vi "Lockin.DAQ.TestLauncher.vi"() -> ()   [LabVIEW 2019, in "Lockin.DAQ.lvclass"]
uses:
  Lockin.DAQ.lvclass
  <vilib>/JKI/JKI SMO/SMO/SMO.lvclass
  <vilib>/JKI/JKI SMO/SMO/Typedefs/SMOState --Enum.ctl
  Typedefs/Set State-enum.ctl
  Instrument.Lockin/Instrument.Lockin.lvclass
  C:/Program Files (x86)/National Instruments/LabVIEW 2016/vi.lib/JKI/JKI SMO/SMO/SMO.lvclass
  Instrument.Lockin/Typedefs/Results Type--Enum.ctl
  Typedefs/Function-enum.ctl
  Typedefs/AO-cluster.ctl
  Typedefs/REF-cluster.ctl
  Typedefs/446xAO-enum.ctl
  Typedefs/AO.config(UI)-cluster.ctl
  Typedefs/AO.config(UI)-array.ctl
  Typedefs/AI.coupling-enum.ctl
  Typedefs/446xAI-enum.ctl
  Typedefs/AI.config(UI)-cluster.ctl
  Typedefs/AI.config(UI)-array.ctl
  Typedefs/Sampling.ctl
  Typedefs/Sample Mode--Ring.ctl
  Typedefs/State-enum.ctl
  Instrument.Lockinl.UI/Typedefs/REF Channel--Cluster.ctl
  Instrument.Lockinl.UI/Instrument.Lockin.UI.lvclass
  Instrument.Lockinl.UI/Typedefs/AO Channel--Cluster.ctl
panel:
  out "DAQ state":T1=enum."created"
  in  "Tab Control 2":T2(tab)=enum."AI"
  out "AO":waveform(dbl)[](graph)
  out "AI":waveform(dbl)[](graph)
  out "WFM 3":waveform(dbl)[](graph)
  out "REF":waveform(dbl)[](graph)
  out "Results":dbl[](graph)
  in  "Reset DAQ":bool
  in  "Stop DAQ":bool
  in  "Start DAQ":bool
  in  "Tab Control":enum32{"Output", "REF", "DAQ"}(tab)=enum."DAQ"
  in  "Channels: AO":T3 {"Phase" format="%.3g"; "Frequency" min=0.0001 max=10000.0 format="%.3g"; "Offset" format="%.3p"; "Amplitude" min=0.0 max=10.0 format="%.3p"}
  in  "Channels: Lockin":T6=[{"Enable?"=FALSE, "Channel"=13, "Frequency"=0.1, "Phase"=0.0, "TC"=1e-05, "Roll-Off"=1}] {"Roll-Off" min=1; "TC" min=0.0001 format="%#_3p"; "Phase" format="%.3g"; "Frequency" min=0.0001 max=10000.0 format="%.3g"}
  in  "Gain":dbl[](array[numeric])=[1.0, 1.0]
  in  "AO Configuration":T8=[{"AO.Range"=enum."±0.1", "AO.channels"="PXI1Slot2/ao0:1"}]
  in  "AI Configuration":T11=[{"AI.Coupling"=10050, "AI.channels"="PXI1Slot2/ai0:1", "AI.Range"=enum."±0.316"}] {"AI.Coupling" items=["AC"=10045, "DC"=10050, "GND"=10066]}
  in  "sampling":T15={"Fs"=204789.0, "#s"=15753}
  in  "sample mode":T16=10123 items=["Finite Samples"=10178, "Continuous Samples"=10123]
  out "SMO State":T17=enum."Stopped"
  out "error out":errorcluster
  in  "Stop":bool
  # "Basic SMO Test Launcher"
  # "For instructions on how to use the JKI State Machine Objects, examples and video tutorials, visit:\nhttp://jki.net/state-machine-objects/\n\nJKI State Machine Objects™\nhttp://jki.net/state-machine-objects/\nCopyright (C) 2005-2015, JKI <info@jki.net>\nALL RIGHTS RESERVED"
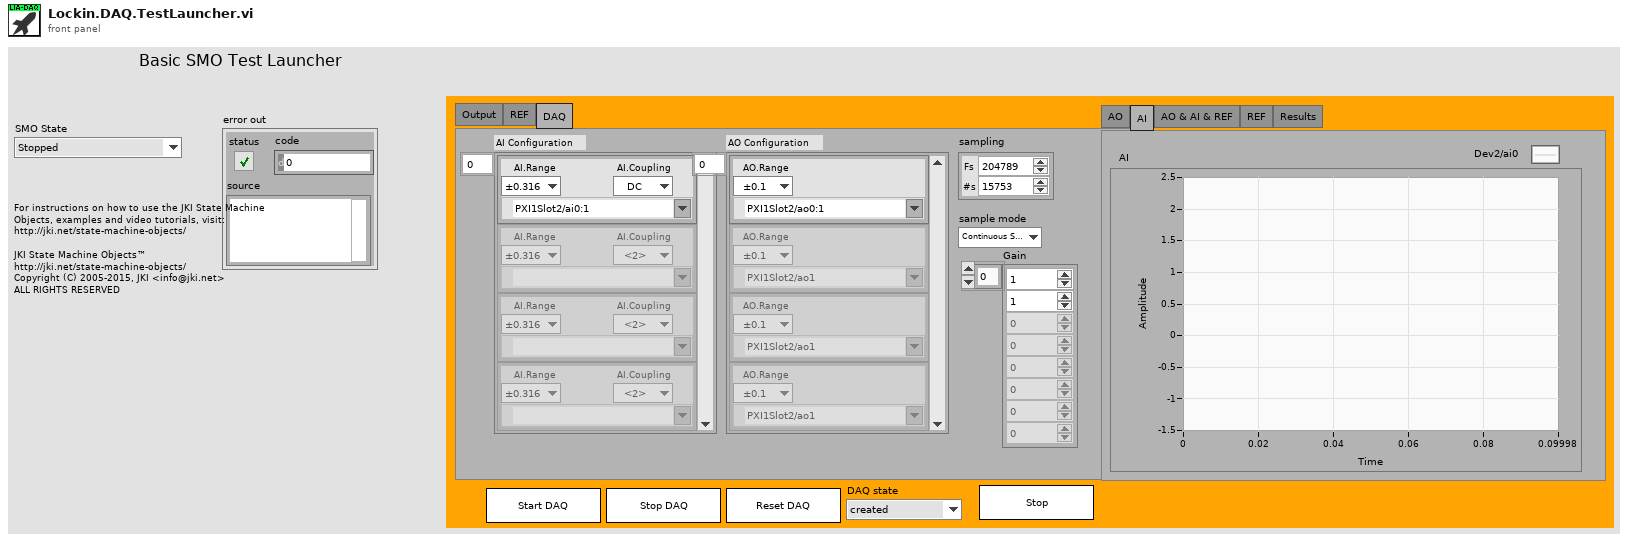
[diagram p1: front panel]
types:
  T1 = typedef "Lockin.DAQ.lvclass/State-enum.ctl" = enum16{"idle", "created", "started", "stopped", "sweeping"}
  T2 = enum32{"AO", "AI", "AO & AI & REF", "REF", "Results"}
  T3 = typedef "Lockin.DAQ.lvclass/AO-cluster.ctl" = T4[]
  T4 = typedef "Instrument.Lockin.UI.lvclass/AO Channel--Cluster.ctl" = cluster{"Enable?":bool, "Channel":i32, "Amplitude":dbl, "Offset":dbl, "Frequency":dbl, "Phase":dbl, "Function":T5, "Sweeping?":bool}
  T5 = typedef "Lockin.DAQ.lvclass/Function-enum.ctl" = enum16{"Sine", "Triangle", "Square"}
  T6 = typedef "Lockin.DAQ.lvclass/REF-cluster.ctl" = T7[]
  T7 = typedef "Instrument.Lockin.UI.lvclass/REF Channel--Cluster.ctl" = cluster{"Enable?":bool, "Channel":i32, "Frequency":dbl, "Phase":dbl, "TC":dbl, "Roll-Off":i32}
  T8 = typedef "Lockin.DAQ.lvclass/AO.config(UI)-array.ctl" = T9[]
  T9 = typedef "Lockin.DAQ.lvclass/AO.config(UI)-cluster.ctl" = cluster{"AO.Range":T10, "AO.channels":tag}
  T10 = typedef "Lockin.DAQ.lvclass/446xAO-enum.ctl" = enum16{"±0.1", "±1.0", "±10.0"}
  T11 = typedef "Lockin.DAQ.lvclass/AI.config(UI)-array.ctl" = T12[]
  T12 = typedef "Lockin.DAQ.lvclass/AI.config(UI)-cluster.ctl" = cluster{"AI.Coupling":T13, "AI.channels":tag, "AI.Range":T14}
  T13 = typedef "Lockin.DAQ.lvclass/AI.coupling-enum.ctl" = u16
  T14 = typedef "Lockin.DAQ.lvclass/446xAI-enum.ctl" = enum16{"±0.316", "±1.00", "±3.16", "±10.0", "±31.6", "±42.4"}
  T15 = typedef "Lockin.DAQ.lvclass/Sampling.ctl" = cluster{"Fs":dbl, "#s":i32}
  T16 = typedef "Lockin.DAQ.lvclass/Sample Mode--Ring.ctl" = i32
  T17 = typedef "SMO.lvclass/SMOState --Enum.ctl" = enum16{"unknown", "Created", "Started", "Stopped"}
  T18 = typedef "SMO.lvclass/Public Events.ctl" = cluster{"Error":refnum<user-event>, "State":refnum<user-event>, "Reserve State":refnum<user-event>}
  T19 = typedef "Lockin.DAQ.lvclass/PublicEvents--Cluster.ctl" = cluster{"getAO":refnum<user-event>, "getAI":refnum<user-event>, "getREF":refnum<user-event>, "getResults":refnum<user-event>, "getCalibration":refnum<user-event>, "getAOChannels":refnum<user-event>, "getREFChannels":refnum<user-event>, "getDAQState":refnum<user-event>, "getSweepResults":refnum<user-event>, "getSweepWaveforms":refnum<user-event>, "getDAQconfig":refnum<user-event>}
  T20 = cluster{"Event Registration Refnum":refnum<event-registration>}
  T21 = typedef "Lockin.DAQ.lvclass/Set State-enum.ctl" = enum16{"start", "stop", "reset", "start sweep", "stop sweep"}
  T22 = typedef "Instrument.Lockin.lvclass/Results Type--Enum.ctl" = enum16{"X", "Y", "R", "Theta", "Mean"}
  T23 = typedef "Lockin.DAQ.lvclass/AI.config-array.ctl" = T24[]
  T24 = typedef "Lockin.DAQ.lvclass/AI.config-cluster.ctl" = cluster{"AI.channels":tag, "AI.Coupling":T13, "AI.Range":T14, "input terminal configuration":i32, "DAQ Type":T25}
  T25 = typedef "Lockin.DAQ.lvclass/DAQType-enum.ctl" = enum16{"None", "USB 4431", "PXI 446x"}
  T26 = typedef "Lockin.DAQ.lvclass/AO.config-array.ctl" = T27[]
  T27 = typedef "Lockin.DAQ.lvclass/AO.config-cluster.ctl" = cluster{"AO.channels":tag, "AO.Range":T10, "output terminal configuration":i32, "DAQ Type":T25}
  T28 = typedef "Lockin.DAQ.lvclass/PublicEvents--Lockin.DAQ.getAO.ctl" = waveform(dbl)[]
  T29 = typedef "Lockin.DAQ.lvclass/PublicEvents--Lockin.DAQ.getAI.ctl" = waveform(dbl)[]
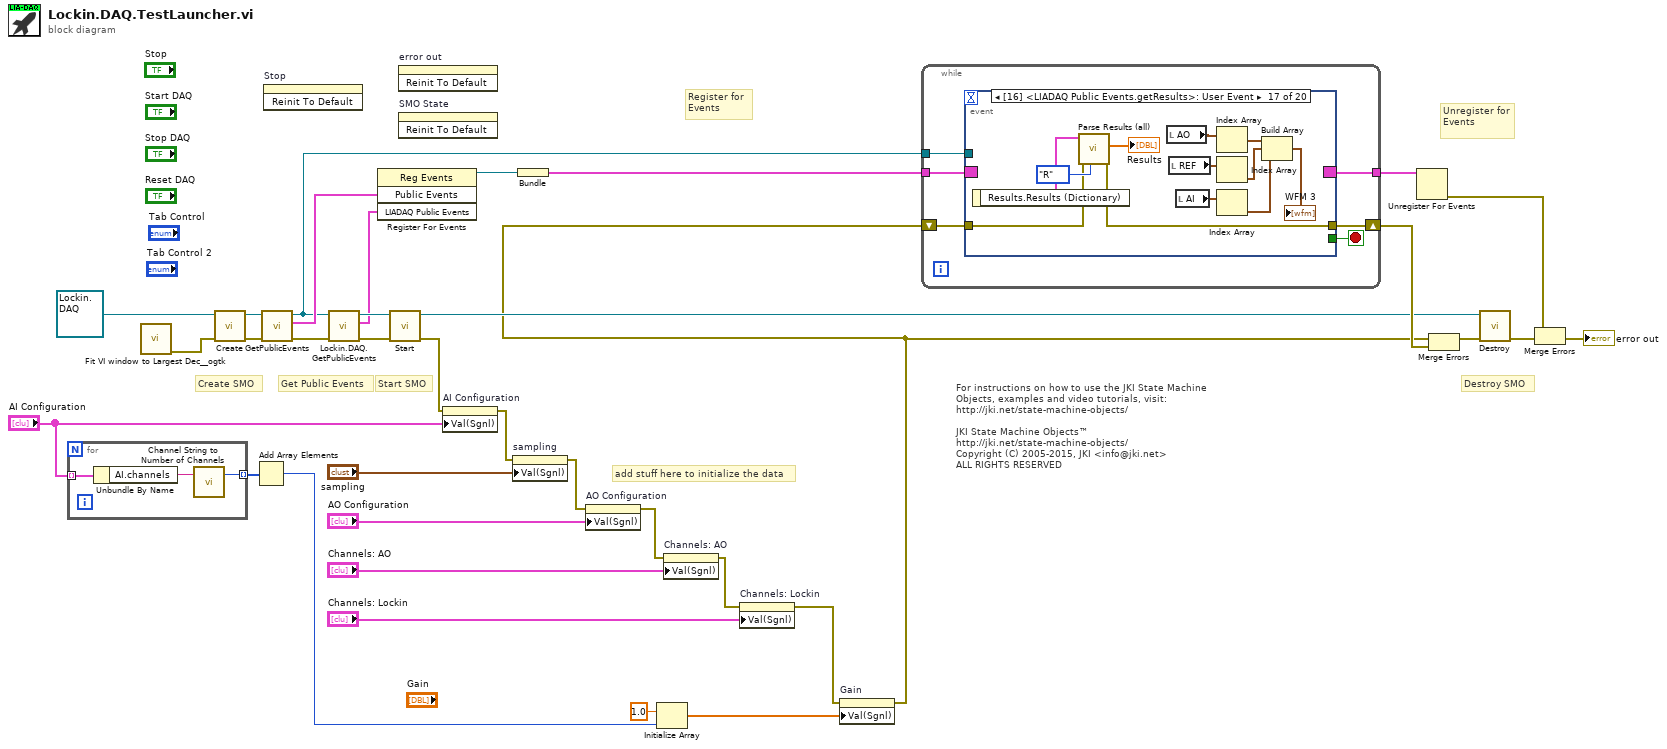
[diagram p0: block diagram]
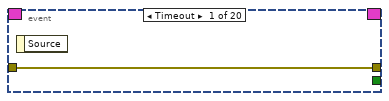
[diagram p2: hidden frame]
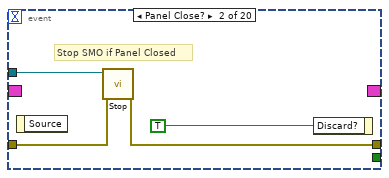
[diagram p3: hidden frame]
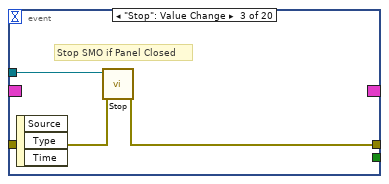
[diagram p4: hidden frame]
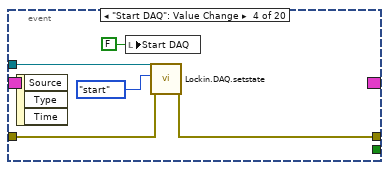
[diagram p5: hidden frame]
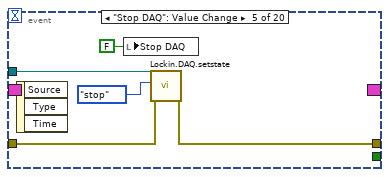
[diagram p6: hidden frame]
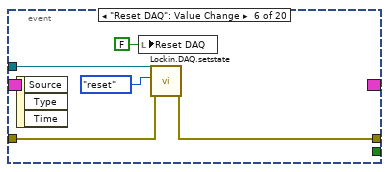
[diagram p7: hidden frame]
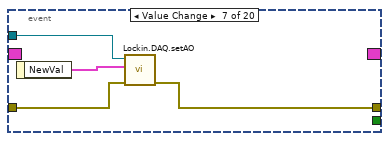
[diagram p8: hidden frame]
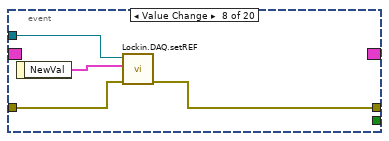
[diagram p9: hidden frame]
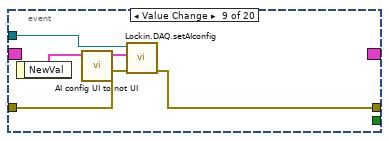
[diagram p10: hidden frame]
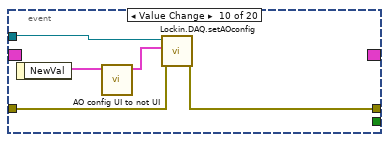
[diagram p11: hidden frame]
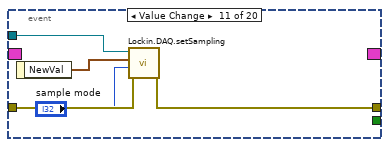
[diagram p12: hidden frame]
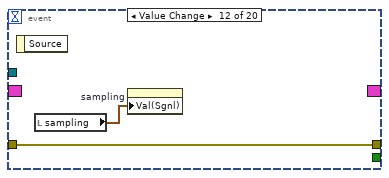
[diagram p13: hidden frame]
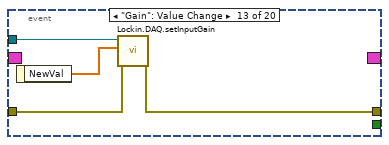
[diagram p14: hidden frame]
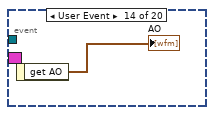
[diagram p15: hidden frame]
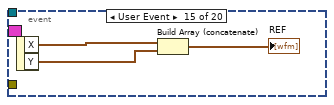
[diagram p16: hidden frame]
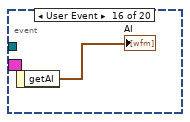
[diagram p17: hidden frame]
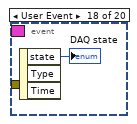
[diagram p18: hidden frame]
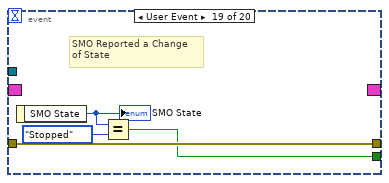
[diagram p19: hidden frame]
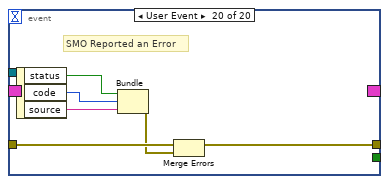
[diagram p20: hidden frame]
diagram:
  # "add stuff here to initialize the data"
  # "For instructions on how to use the JKI State Machine Objects, examples and video tutorials, visit:\nhttp://jki.net/state-machine-objects/\n\nJKI State Machine Objects™\nhttp://jki.net/state-machine-objects/\nCopyright (C) 2005-2015, JKI <info@jki.net>\nALL RIGHTS RESERVED"
  # "Get Public Events"
  # "Start SMO"
  # "Destroy SMO"
  # "Create SMO"
  # "Unregister for Events"
  # "Register for Events"
  n1 = for {
    tunnel: "AI Configuration" -> [w38] mode=indexing
    tunnel: [w36] -> w8 mode=indexing
    n2 = Unbundle By Name(w38) -> ("AI.channels"=w37:tag)
    n3 = call "Channel String to Number of Channels.vi"("Channels String"=w37) -> ("# channels"=w36:i32)  [unwired: 2 in]
  }
  n4 = call <userlib>:"Fit VI window to Largest Dec__ogtk.vi"() -> ("error out"=w1:errorcluster)  [unwired: 6 in, 1 out]
  n5 = call <vilib>:"Create.vi"("error in (no error)"=w1, "SMO"=refnum<class "Lockin.DAQ.lvclass"> refnum ("Lockin.DAQ.lvclass")) -> ("error out"=w27:errorcluster, "SMO out"=w28:refnum<class "Lockin.DAQ.lvclass">)  [unwired: 7 in, 1 out]
  n6 = Add Array Elements(numeric array=w8) -> (sum=w5:i32)
  n7 = call <vilib>:"GetPublicEvents.vi"("error in (no error)"=w27, "SMO"=w28) -> ("error out"=w24:errorcluster, "Public Events"=w26:T18, "SMO out"=w23:refnum<class "Lockin.DAQ.lvclass">)  [unwired: 7 in]
  n8 = invoke on="Stop" class="Bool" method="Reinit To Default"() -> ()  [unwired: 3 in, 3 out]
  n9 = call "Lockin.DAQ.GetPublicEvents.vi"("error in (no error)"=w24, "Lockin.DAQ"=w23) -> ("error out"=w21:errorcluster, "LIADAQ Public Events"=w20:T19, "Lockin.DAQ out"=w22:refnum<class "Lockin.DAQ.lvclass">)  [unwired: 7 in]
  n10 = register-events(w26, w20) -> (reference out=w25:refnum<event-registration>)  [unwired: 2 in, 1 out]
  n11 = call <vilib>:"Start.vi"("error in (no error)"=w21, "SMO"=w22) -> ("error out"=w10:errorcluster, "SMO out"=w11:refnum<class "Lockin.DAQ.lvclass">)  [unwired: 8 in]
  n12 = invoke on="error out" class="Clust (strict)" method="Reinit To Default"() -> ()  [unwired: 3 in, 3 out]
  n13 = invoke on="SMO State" class="Enum (strict)" method="Reinit To Default"() -> ()  [unwired: 3 in, 3 out]
  n14 = property on="AI Configuration" class="Arr (strict)"(error in=w10, "Val(Sgnl)"="AI Configuration") -> (error out=w13:errorcluster)  [unwired: 1 in, 1 out]
  n15 = property on="sampling" class="Clust (strict)"(error in=w13, "Val(Sgnl)"="sampling") -> (error out=w14:errorcluster)  [unwired: 1 in, 1 out]
  n16 = Bundle("Event Registration Refnum"=w25) -> (w34:T20)  [unwired: 1 in]
  n17 = property on="AO Configuration" class="Arr (strict)"(error in=w14, "Val(Sgnl)"="AO Configuration") -> (error out=w15:errorcluster)  [unwired: 1 in, 1 out]
  n18 = Initialize Array(1.0 ("element"), w5) -> (w6:dbl[])
  n19 = property on="Channels: AO" class="Arr (strict)"(error in=w15, "Val(Sgnl)"="Channels: AO") -> (error out=w12:errorcluster)  [unwired: 1 in, 1 out]
  n20 = property on="Channels: Lockin" class="Arr (strict)"(error in=w12, "Val(Sgnl)"="Channels: Lockin") -> (error out=w3:errorcluster)  [unwired: 1 in, 1 out]
  n21 = property on="Gain" class="Arr (strict)"(error in=w3, "Val(Sgnl)"=w6) -> (error out=w4:errorcluster)  [unwired: 1 in, 1 out]
  n22 = while {
    shift-right: [w43] -> w33
    shift-left: w4 -> [w42]
    tunnel: w34 -> [w41]
    tunnel: [w40] -> w35
    tunnel: w23 -> [w39]
    stop <- w44 stop-if-true
    n23 = event shown="[16] <LIADAQ Public Events.getResults>: User Event" {
      selector: w41 -> [_ _ _ _ _ _ _ _ _ _ _ _ _ _ _ _ _ _ _ _]
      dyn-events: [_ _ _ _ _ _ _ _ _ _ _ _ _ _ _ _ _ _ _ _] -> w40
      timeout: _ -> [_ _ _ _ _ _ _ _ _ _ _ _ _ _ _ _ _ _ _ _]
      tunnel: [_ _ _ _ _ _ _ _ _ _ _ _ _ _ _ _ _ _ w115 _] -> w44
      tunnel: w39 -> [_ w49 w52 w57 w62 w67 w70 w74 w80 w81 w90 _ w96 _ _ _ _ _ _ _]
      tunnel: [w45 w48 w51 w56 w61 w66 w68 w72 w78 w82 w88 w91 w94 _ _ _ w102 _ w118 w122] -> w43
      tunnel: w42 -> [w45 w47 w50 w55 w60 w65 w69 w73 w79 w83 w89 w91 w95 _ _ _ w103 _ w118 w120]
      event Timeout {
        n24 = event-data() -> ()  [unwired: 1 in, 1 out]
      }
      event Panel Close? {
        # "Stop SMO if Panel Closed"
        n25 = event-data() -> ()  [unwired: 1 in, 1 out]
        n26 = call <vilib>:"Stop.vi"("error in (no error)"=w47, "SMO"=w49) -> ("error out"=w48:errorcluster)  [unwired: 8 in, 1 out]
        n27 = event-data("Discard?"=TRUE ("OK")) -> ()  [unwired: 1 in, 1 out]
      }
      event "Stop": Value Change {
        # "Stop SMO if Panel Closed"
        n28 = event-data() -> ()  [unwired: 1 in, 3 out]
        n29 = call <vilib>:"Stop.vi"("error in (no error)"=w50, "SMO"=w52) -> ("error out"=w51:errorcluster)  [unwired: 8 in, 1 out]
      }
      event "Start DAQ": Value Change {
        n30 = event-data() -> ()  [unwired: 1 in, 3 out]
        n31 = local write "Start DAQ"(FALSE ("Start DAQ")) -> ()
        n32 = call "Lockin.DAQ.setstate.vi"("error in (no error)"=w55, "State"=Set_State-enum."start" ("setState"), "Lockin.DAQ"=w57) -> ("error out"=w56:errorcluster)  [unwired: 7 in, 1 out]
      }
      event "Stop DAQ": Value Change {
        n33 = event-data() -> ()  [unwired: 1 in, 3 out]
        n34 = local write "Stop DAQ"(FALSE ("Stop DAQ")) -> ()
        n35 = call "Lockin.DAQ.setstate.vi"("error in (no error)"=w60, "State"=Set_State-enum."stop" ("setState"), "Lockin.DAQ"=w62) -> ("error out"=w61:errorcluster)  [unwired: 7 in, 1 out]
      }
      event "Reset DAQ": Value Change {
        n36 = event-data() -> ()  [unwired: 1 in, 3 out]
        n37 = local write "Reset DAQ"(FALSE ("Reset DAQ")) -> ()
        n38 = call "Lockin.DAQ.setstate.vi"("error in (no error)"=w65, "State"=Set_State-enum."reset" ("setState"), "Lockin.DAQ"=w67) -> ("error out"=w66:errorcluster)  [unwired: 7 in, 1 out]
      }
      event Value Change {
        n39 = event-data() -> ("NewVal"=w71:T3)  [unwired: 1 in]
        n40 = call "Lockin.DAQ.setAO.vi"("error in (no error)"=w69, "AO Channels"=w71, "Lockin.DAQ"=w70) -> ("error out"=w68:errorcluster)  [unwired: 7 in, 1 out]
      }
      event Value Change {
        n41 = event-data() -> ("NewVal"=w75:T6)  [unwired: 1 in]
        n42 = call "Lockin.DAQ.setREF.vi"("error in (no error)"=w73, "Channels: Lockin"=w75, "Lockin.DAQ"=w74) -> ("error out"=w72:errorcluster)  [unwired: 7 in, 1 out]
      }
      event Value Change {
        n43 = event-data() -> ("NewVal"=w77:T11)  [unwired: 1 in]
        n44 = call "AI config UI to not UI.vi"("AI Config (UI)"=w77) -> ("AI Config"=w76:T23)  [unwired: 10 in]
        n45 = call "Lockin.DAQ.setAIconfig.vi"("error in (no error)"=w79, "AI Configuration"=w76, "Lockin.DAQ"=w80) -> ("error out"=w78:errorcluster)  [unwired: 7 in, 1 out]
      }
      event Value Change {
        n46 = event-data() -> ("NewVal"=w85:T8)  [unwired: 1 in]
        n47 = call "AO config UI to not UI.vi"("AO Config (UI)"=w85) -> ("AO Config"=w84:T26)  [unwired: 10 in]
        n48 = call "Lockin.DAQ.setAOconfig.vi"("error in (no error)"=w83, "AO Configuration"=w84, "Lockin.DAQ"=w81) -> ("error out"=w82:errorcluster)  [unwired: 7 in, 1 out]
      }
      event Value Change {
        n49 = event-data() -> ("NewVal"=w87:T15)  [unwired: 1 in]
        n50 = call "Lockin.DAQ.setSampling.vi"("error in (no error)"=w89, "Sample Mode"="sample mode", "Sampling"=w87, "Lockin.DAQ"=w90) -> ("error out"=w88:errorcluster)  [unwired: 6 in, 1 out]
      }
      event Value Change {
        n51 = event-data() -> ()  [unwired: 1 in, 1 out]
        n52 = local read "sampling"() -> (w92:T15)
        n53 = property on="sampling" class="Clust (strict)"("Val(Sgnl)"=w92) -> ()  [unwired: 2 in, 2 out]
      }
      event "Gain": Value Change {
        n54 = event-data() -> ("NewVal"=w93:dbl[])  [unwired: 1 in]
        n55 = call "Lockin.DAQ.setInputGain.vi"("error in (no error)"=w95, "setInputGain"=w93, "Lockin.DAQ"=w96) -> ("error out"=w94:errorcluster)  [unwired: 7 in, 1 out]
      }
      event User Event {
        n56 = event-data() -> ("get AO"=→"AO":T28)  [unwired: 1 in]
      }
      event User Event {
        n57 = event-data() -> ("X"=w99:waveform(dbl)[], "Y"=w98:waveform(dbl)[])  [unwired: 1 in]
        n58 = Build Array (concatenate)(w99, w98) -> (→"REF":waveform(dbl)[])
      }
      event User Event {
        n59 = event-data() -> ("getAI"=→"AI":T29)  [unwired: 1 in]
      }
      event User Event {
        n60 = event-data() -> ("Results.Results (Dictionary)"=w106:cluster{"key":string, "value":dbl}[])  [unwired: 1 in]
        n61 = call "Parse Results (all).vi"("Type"=Results_Type--Enum."R", "error in (no error)"=w103, "Results (Dictionary)"=w106) -> ("error out"=w102:errorcluster, "Data"=→"Results":dbl[])  [unwired: 5 in, 2 out]
        n62 = local read "AO"() -> (w113:waveform(dbl)[])
        n63 = local read "REF"() -> (w112:waveform(dbl)[])
        n64 = local read "AI"() -> (w111:waveform(dbl)[])
        n65 = Index Array(array=w113) -> (element=w110:waveform(dbl))  [unwired: 1 in]
        n66 = Index Array(array=w112) -> (element=w109:waveform(dbl))  [unwired: 1 in]
        n67 = Index Array(array=w111) -> (element=w107:waveform(dbl))  [unwired: 1 in]
        n68 = Build Array(w110, w109, w107) -> (→"WFM 3":waveform(dbl)[])
      }
      event User Event {
        n69 = event-data() -> ("state"=→"DAQ state":T1)  [unwired: 1 in, 2 out]
      }
      event User Event {
        # "SMO Reported a Change\nof State"
        n70 = event-data() -> ("SMO State"=w117:T17)  [unwired: 1 in]
        "SMO State" <- w117
        n71 = Equal?(x=w117, y=SMOState_--Enum."Stopped") -> (x = y?=w115:bool)
      }
      event User Event {
        # "SMO Reported an Error"
        n72 = event-data() -> ("status"=w121:bool, "code"=w124:i32, "source"=w123:string)  [unwired: 1 in]
        n73 = Bundle("status"=w121, "code"=w124, "source"=w123) -> (w119:errorcluster)  [unwired: 1 in]
        n74 = Merge Errors(w120, w119) -> (w122:errorcluster)
      }
    }
  }
  n75 = Unregister For Events(event registration refnum=w35) -> (error out=w32:errorcluster)  [unwired: 1 in]
  n76 = Merge Errors(w4, w33) -> (w29:errorcluster)
  n77 = call <vilib>:"Destroy.vi"("error in (no error)"=w29, "SMO"=w11) -> ("error out"=w30:errorcluster)  [unwired: 9 in]
  n78 = Merge Errors(w32, w30) -> (→"error out":errorcluster)
